vi "StopData.vi"(8 "error in (no error)":errorcluster, 11 "Class In":refnum<class "C37.118 PMU.lvclass">) -> (0 "error out":errorcluster, 3 "Class Out":refnum<class "C37.118 PMU.lvclass">)   [LabVIEW 2018, in "SensorPlugins.lvlib" / "C37.118 PMU.lvclass"]
uses:
  C37.118 PMU.lvclass
  Typedef/eCmdTypes.ctl
  C37.118 PMU.lvclass/C37.118 PMU.ctl
  Accessors/Read CmdSocket.vi
  Accessors/Read PMUComms.vi
  Accessors/Read DataSocket.vi
  Accessors/Write CmdSocket.vi
  Accessors/Write DataSocket.vi
  <userlib>/NIST/Socket Class/Classes/Socket.Base/Socket.Base.lvclass
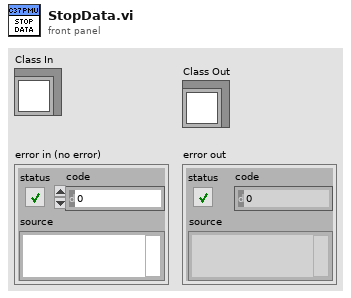
[diagram p1: front panel]
types:
  T1 = typedef "SensorPlugins.lvlib/C37.118 PMU.lvclass/eCmdTypes.ctl" = enum16{"Stop realtime data", "Start realtime data", "Send HDR file", "Send CFG-1 file", "Send CFG-2 file"}
  T2 = typedef "SensorPlugins.lvlib/C37.118 PMU.lvclass/PMUComms.ctl" = cluster{"PMU IP Address":string, "CMD Comms Type":T3, "Data Comms Type":T3, "CMD Port":u16, "Data Port":u16, "PMU ID":u16}
  T3 = typedef "SensorPlugins.lvlib/C37.118 PMU.lvclass/eCommsType.ctl" = enum16{"TCP", "UDP", "USB", "GPIB"}
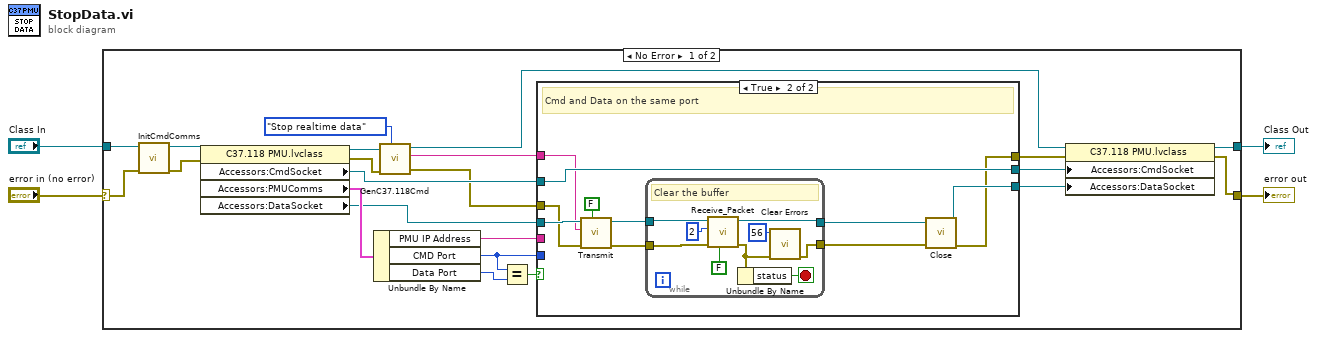
[diagram p0: block diagram]
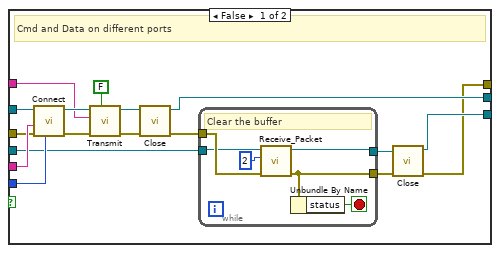
[diagram p2: hidden frame]
diagram:
  n1 = case shown="No Error" "error in (no error)" {
    selector: "error in (no error)" -> [w14 w70]
    tunnel: "Class In" -> [w16 w71]
    tunnel: [w20 w71] -> w2
    tunnel: [w18 w70] -> w1
    frame No Error {
      n2 = call "InitCmdComms.vi"("error in (no error)"=w14, "C37.118 PMU in"=w16) -> ("error out"=w13:errorcluster, "C37.118 PMU out"=w15:refnum<class "C37.118 PMU.lvclass">)  [unwired: 8 in]
      n3 = property class="C37.118 PMU.lvclass"(reference=w15, error in=w13) -> (reference out=w25:refnum<class "C37.118 PMU.lvclass">, error out=w12:errorcluster, "Accessors:CmdSocket"=w24:refnum<class "Socket.Base.lvclass">, "Accessors:PMUComms"=w23:T2, "Accessors:DataSocket"=w7:refnum<class "Socket.Base.lvclass">)
      n4 = Unbundle By Name(w23) -> ("PMU IP Address"=w22:string, "CMD Port"=w10:u16, "Data Port"=w11:u16)
      n5 = call "GenC37.118Cmd.vi"("Function"=eCmdTypes."Stop realtime data", "error in (no error)"=w12, "PMUClass"=w25) -> ("error out"=w5:errorcluster, "Command"=w21:string, "PMUClass"=w9:refnum<class "C37.118 PMU.lvclass">)  [unwired: 6 in]
      n6 = Equal?(x=w10, y=w11) -> (x = y?=w8:bool)
      n7 = case shown="True" w8 {
        tunnel: w24 -> [w43 w60]
        tunnel: w22 -> [w42 _]
        tunnel: w21 -> [w38 w57]
        tunnel: [w35 w60] -> w19
        tunnel: [w28 w50] -> w17
        tunnel: w10 -> [w34 _]
        tunnel: w7 -> [w32 w58]
        tunnel: [w29 w51] -> w6
        tunnel: w5 -> [w27 w56]
        frame False {
          # "Cmd and Data on different ports"
          n8 = call-dynamic "Connect.vi"("remote_port"=w34, "error in (no error)"=w27, "remote_address"=w42, "Socket.Base in"=w43) -> ("error out"=w39:errorcluster, "Socket.Base out"=w40:refnum<class "Socket.Base.lvclass">)  [unwired: 6 in]
          n9 = call-dynamic "Transmit.vi"("packet? (f)"=FALSE, "error in (no error)"=w39, "data"=w38, "Socket.Base in"=w40) -> ("error out"=w37:errorcluster, "Socket.Base out"=w36:refnum<class "Socket.Base.lvclass">)  [unwired: 5 in, 1 out]
          n10 = call-dynamic "Close.vi"("error in (no error)"=w37, "Socket.Base in"=w36) -> ("error out"=w33:errorcluster, "Socket.Base out"=w35:refnum<class "Socket.Base.lvclass">)  [unwired: 8 in]
          n11 = while {
            tunnel: w33 -> [w48]
            tunnel: w32 -> [w46]
            tunnel: [w45] -> w31
            tunnel: [w44] -> w30
            stop <- w47 stop-if-true
            # "Clear the buffer"
            n12 = call-dynamic "Receive_Packet.vi"("error in (no error)"=w48, "bufsize (0)"=u32 2, "Socket.Base in"=w46) -> ("error out"=w45:errorcluster, "Socket.Base out"=w44:refnum<class "Socket.Base.lvclass">)  [unwired: 5 in, 2 out]
            n13 = Unbundle By Name(w45) -> ("status"=w47:bool)
          }
          n14 = call-dynamic "Close.vi"("error in (no error)"=w31, "Socket.Base in"=w30) -> ("error out"=w28:errorcluster, "Socket.Base out"=w29:refnum<class "Socket.Base.lvclass">)  [unwired: 8 in]
        }
        frame True {
          # "Cmd and Data on the same port"
          n15 = call-dynamic "Transmit.vi"("packet? (f)"=FALSE, "error in (no error)"=w56, "data"=w57, "Socket.Base in"=w58) -> ("error out"=w54:errorcluster, "Socket.Base out"=w55:refnum<class "Socket.Base.lvclass">)  [unwired: 5 in, 1 out]
          n16 = while {
            tunnel: w54 -> [w68]
            tunnel: w55 -> [w66]
            tunnel: [w62] -> w53
            tunnel: [w64] -> w52
            stop <- w67 stop-if-true
            # "Clear the buffer"
            n17 = call-dynamic "Receive_Packet.vi"("clear_timeout_error (f)"=FALSE, "error in (no error)"=w68, "bufsize (0)"=u32 2, "Socket.Base in"=w66) -> ("error out"=w65:errorcluster, "Socket.Base out"=w64:refnum<class "Socket.Base.lvclass">)  [unwired: 4 in, 2 out]
            n18 = Unbundle By Name(w65) -> ("status"=w67:bool)
            n19 = call <vilib>:"Clear Errors.vi"("error in (no error)"=w65, "specific error code to clear (0: all)"=56) -> ("error out"=w62:errorcluster)  [unwired: 4 in, 1 out]
          }
          n20 = call-dynamic "Close.vi"("error in (no error)"=w53, "Socket.Base in"=w52) -> ("error out"=w50:errorcluster, "Socket.Base out"=w51:refnum<class "Socket.Base.lvclass">)  [unwired: 8 in]
        }
      }
      n21 = property class="C37.118 PMU.lvclass"(reference=w9, error in=w17, "Accessors:CmdSocket"=w19, "Accessors:DataSocket"=w6) -> (reference out=w20:refnum<class "C37.118 PMU.lvclass">, error out=w18:errorcluster)
    }
    frame Error {
    }
  }
  "Class Out" <- w2
  "error out" <- w1
